vi "系统设置.vi"() -> ()   [LabVIEW 2016]
uses:
  <userlib>/_SmartBalloon/Balloon Generic/Aesthetics.ctl
  <vilib>/Utility/miscctls.llb/LVPointTypeDef.ctl
  <userlib>/_SmartBalloon/Balloon/Text Balloon.lvclass
  C:/Program Files (x86)/National Instruments/LabVIEW 2016/user.lib/_SmartBalloon/Balloon Generic/Balloon.lvclass
  <userlib>/_SmartBalloon/Balloon/Init Balloon.vi
  <vilib>/ptbypt/NI_PtbyPt.lvlib
  <vilib>/Utility/config.llb/NI_LVConfig.lvlib
  PLC/PLC.lvlib
  <userlib>/_SmartBalloon/API/SmartBalloon Library.lvclass
  <userlib>/_SmartBalloon/Balloon Generic/Balloon.lvclass
  API/WxMessage/wxpusher.lvlib
panel:
  out "最近一次启动时间":string
  in  "添加防火墙":bool
  in  "系统单次测试":bool
  in  "站点配置":bool
  in  "微信关注扫码":bool
  in  "updateconfiguration":T1={"主机"="27.154.58.30", "用户"="update", "密码"="std23506", "远程路径"="数据传输系统\\平台数据传输系统.exe", "下载文件名"="平台数据传输系统.exe", "软件版本"=""}
  in  "周期运行启动参数":T2
  in  "更新":bool
  in  "模块启用配置":bool
  in  "短信报警设置":bool
  in  "首页显示设置":bool
  in  "跨度核查":bool
  in  "空白核查":bool
  out "选项卡控件":enum32{"自由设定", "国标协议", "流量设定"}(tab)
  in  "24H周期设置":bool[](xcontrol)
  in  "多参数运行间隔":i16=4 min=1 max=24
  in  "运行间隔":i16=4 caption="湿化学运行间隔" min=1 max=24
  in  "流量阈值":dbl=4.0 min=1.0 max=24.0
  in  "时间阈值":u16=4 min=1 max=24
  in  "周期设置":enum16{"自由设定", "国标协议", "流量设定"}(ring)
  out "x = y?":bool
  in  "质控启动日期":string(combo)="关闭"
  in  "跨度核查时间":T3(ring)=enum."06H"
  in  "空白核查时间":T3(ring)=enum."02H"
  in  "输入密码":dbl
  out "布尔":bool
  in  "开机启动":bool caption="氨氮禁用"
  in  "运行模式":enum16{"维护模式", "常规模式", "应急模式", "质控模式"}(ring)
  # "注：周期设置分为自由设定和国标协议两种。\n1：选择自由设定情况下：运行间隔将不可选用并变灰色，周期设置可自由手动勾选\n2：选择国标协议情况下：周期时间将由运行间隔选择的时间决定，下方周期设置被禁用并无法手动勾选。\n3：选择流量设定情况下：瞬时流量连续超过流量阈值到达时间阈值设定值，仪器将自动开启测量。"
  # "质控频次："
  # "零点核查时间："
  # "跨度核查时间："
  # "启动周期设置"
  # "m3/S"
  # "秒"
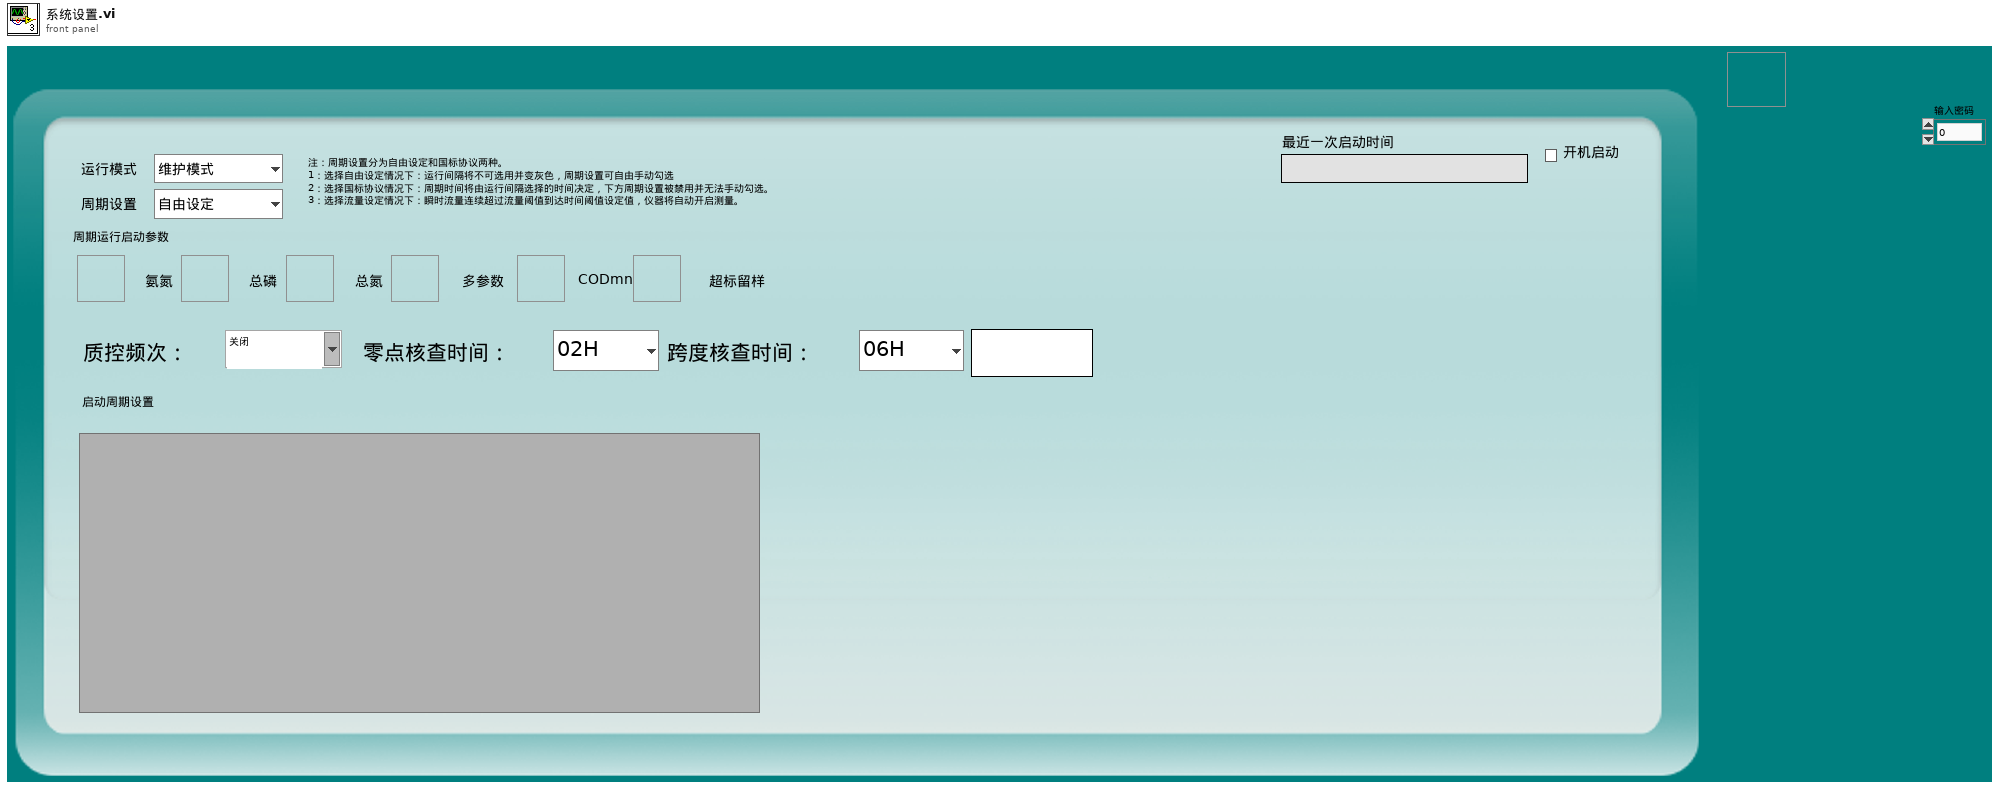
[diagram p1: front panel]
types:
  T1 = cluster{"主机":string, "用户":string, "密码":string, "远程路径":string, "下载文件名":string, "软件版本":string}
  T2 = cluster{"氨氮":bool, "总磷":bool, "总氮":bool, "多参数":bool, "CODmn":bool, "CODCr":bool, "超标留样":bool}
  T3 = enum16{"00H", "01H", "02H", "03H", "04H", "05H", "06H", "07H", "08H", "09H", "10H", "11H", "12H", "13H", "14H", "15H", "16H", "17H", "18H", "19H", "20H", "21H", "22H", "23H", "关闭"}
  T4 = enum16{"启动测量", "标样核查", "零点核查", "跨度核查", "空白测试", "平行样测试", "加标回收", "空白校准", "标样校准", "初始化（清洗）", "停止测试", "仪器重启", "校时", "模式设置", "测量间隔设置"}
  T5 = cluster{"参数启用":cluster{"氨氮":bool, "总磷":bool, "总氮":bool, "多参数":bool, "CODMn":bool, "CODcr":bool, "超标留样":bool}}
  T6 = typedef "LVPointTypeDef.ctl" = cluster{"Horizontal":i16, "Vertical":i16}
  T7 = enum32{"Bad", "Idle", "Run top level", "Running"}
  T8 = typedef "Balloon Engine.lvlib/Balloon.lvclass/Aesthetics.ctl" = cluster{"Colors":cluster{"Font Color":u32, "Panel Color":u32}, "Display Time (ms)":i32}
  T9 = cluster{"运行模式":enum16{"维护模式", "常规模式", "应急模式", "质控模式"}, "质控频次":enum16{"关闭", "每天", "星期一", "星期二", "星期三", "星期四", "星期五", "星期六", "星期日"}, "空白核查时间":u16, "跨度核查时间":u16, "24H周期设置":bool[]}
  T10 = typedef "LVDateTimeRec.ctl" = cluster{"秒数的小数部分":dbl, "秒":i32, "分":i32, "时":i32, "日":i32, "月":i32, "年":i32, "天数（周）":i32, "天数（年）":i32, "DST":i32}
  T11 = enum32{"Invalid", "Standard", "Closed", "Hidden", "Minimized", "Maximized"}
  T12 = typedef "NI_LVConfig.lvlib/Config Data RefNum.ctl" = refnum<k1>
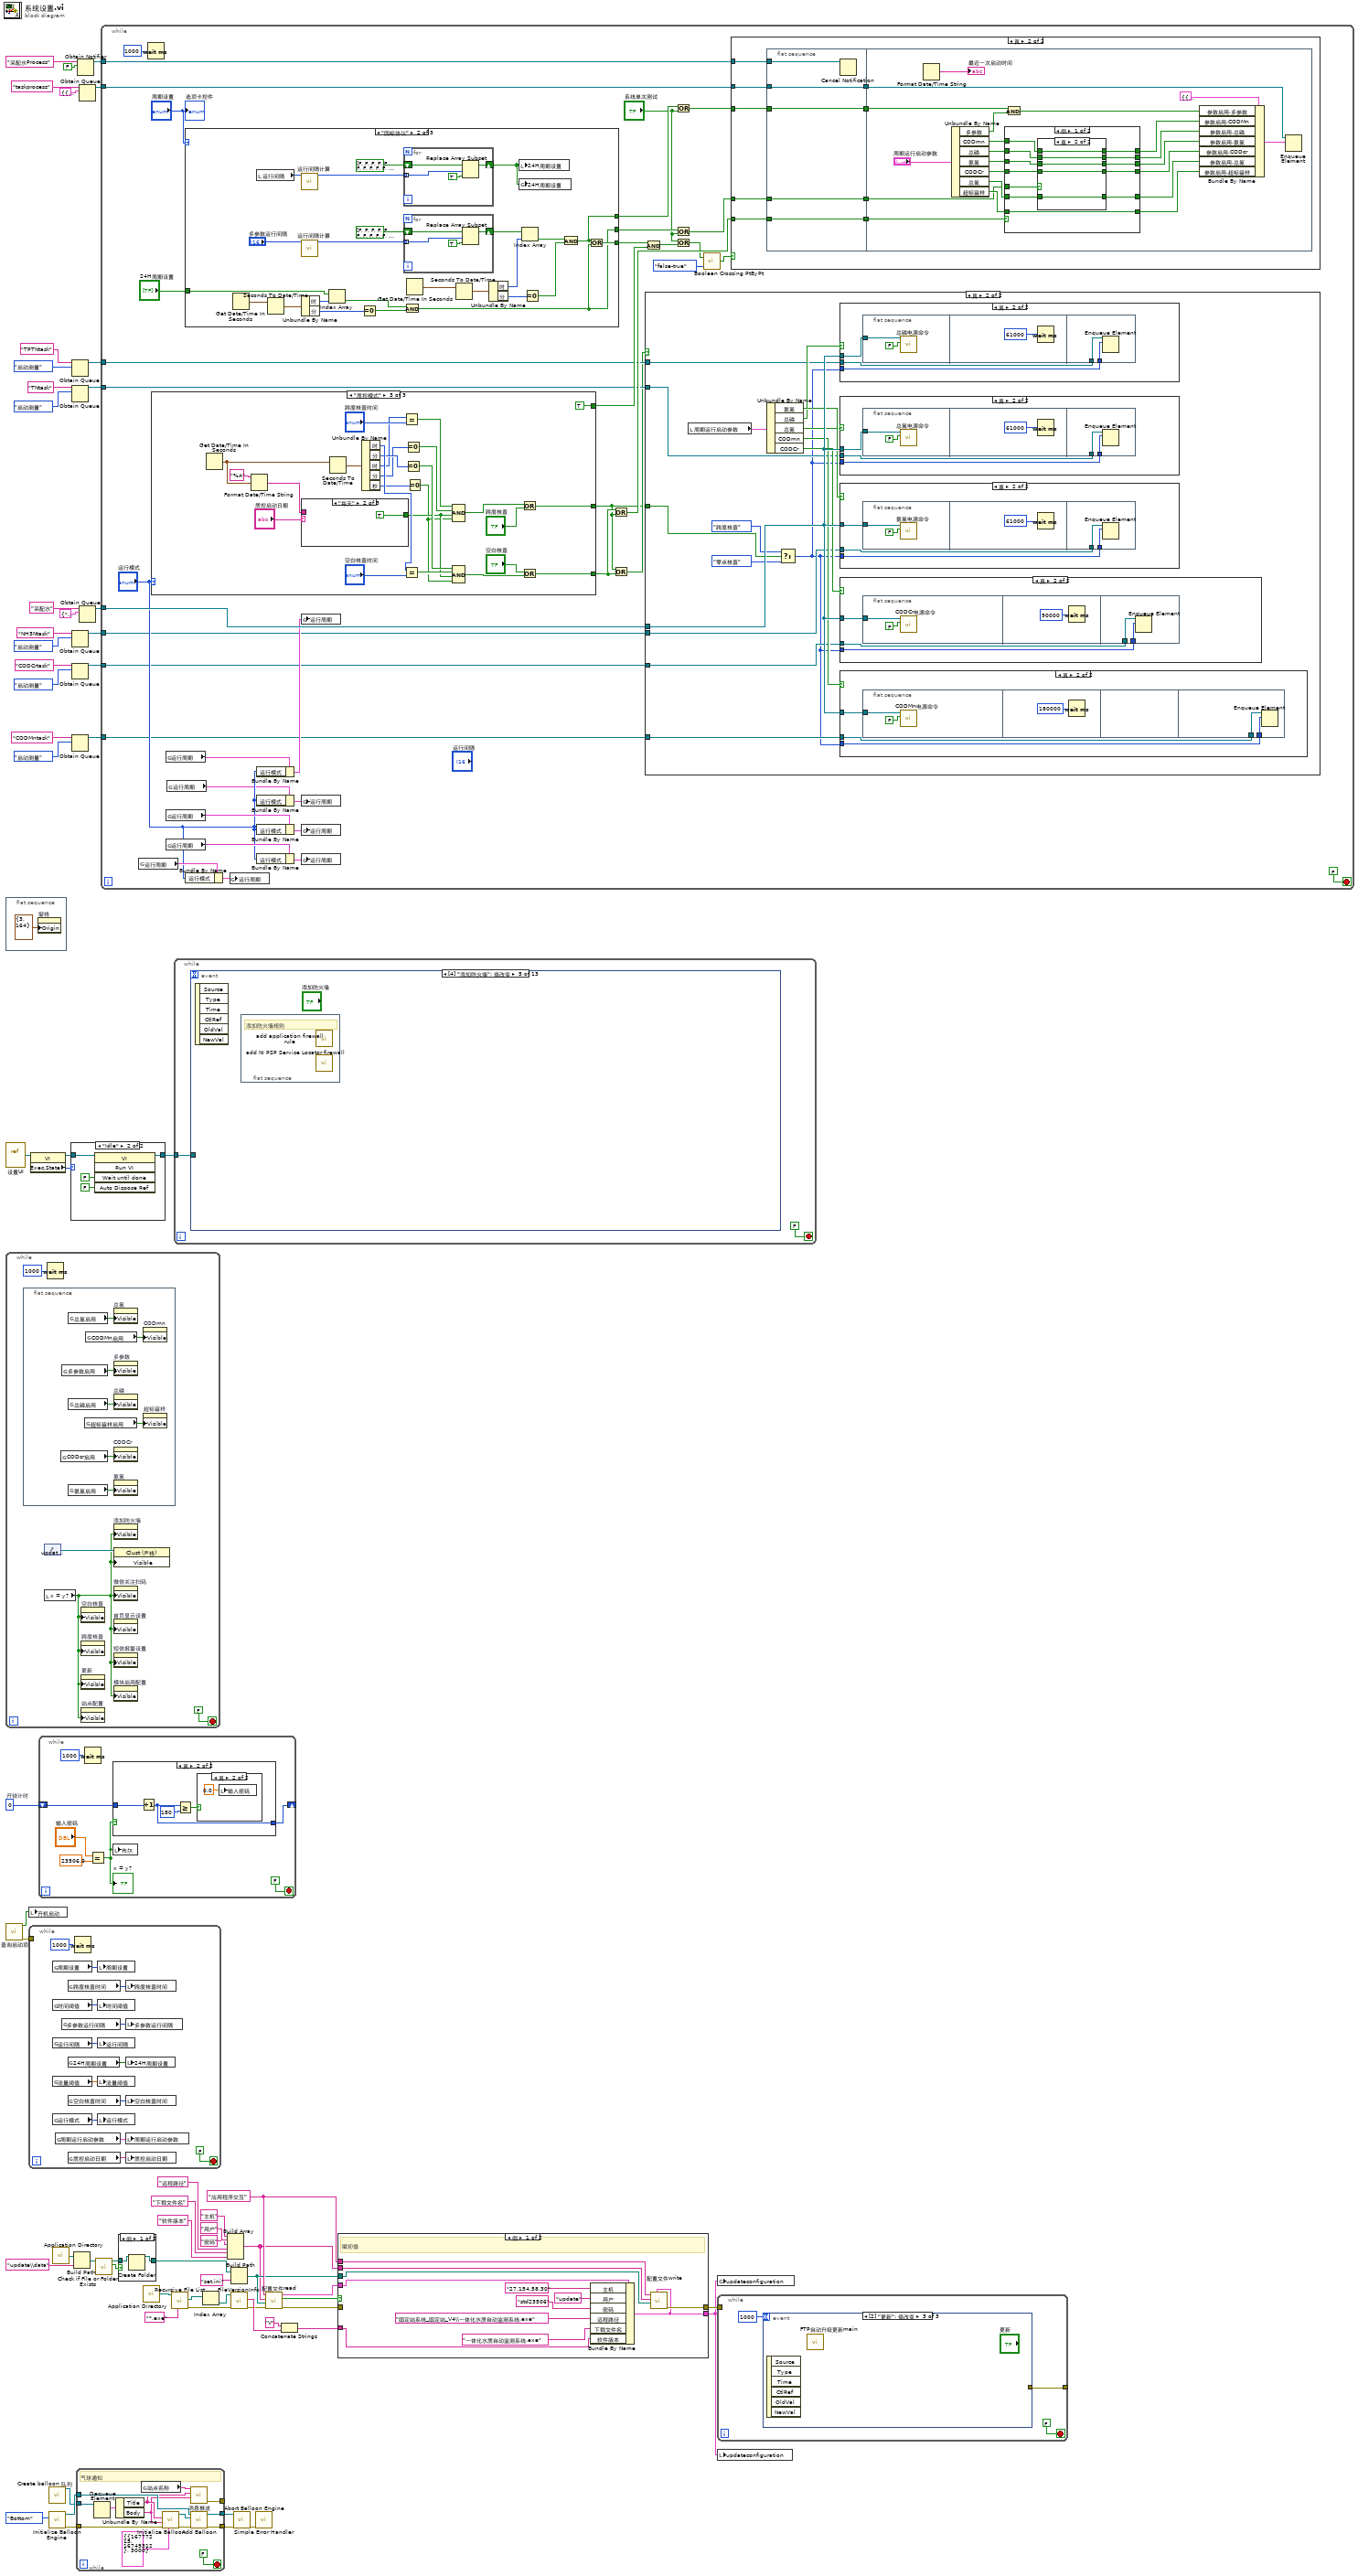
[diagram p0: block diagram]
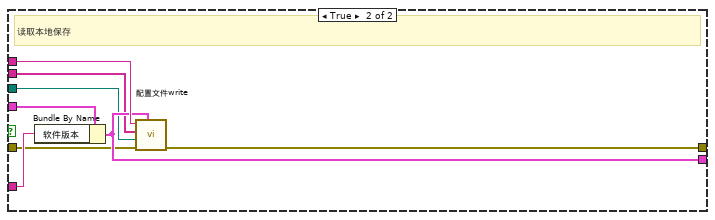
[diagram p3: hidden frame]
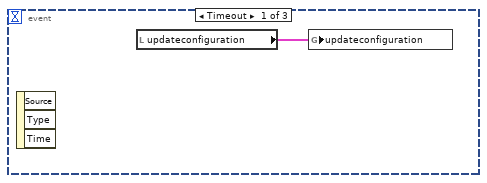
[diagram p4: hidden frame]
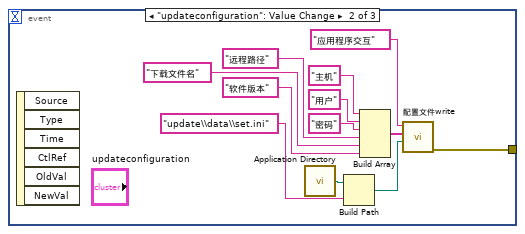
[diagram p5: hidden frame]
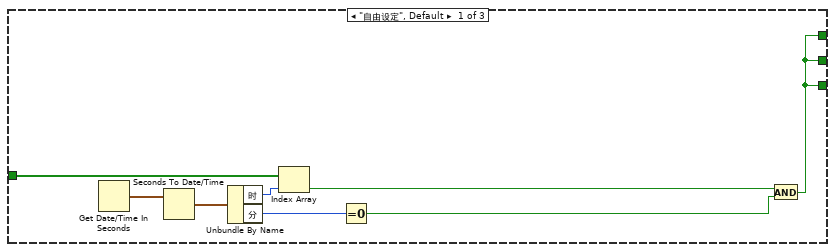
[diagram p9: hidden frame]
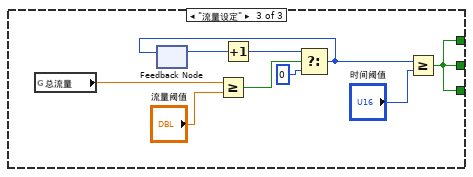
[diagram p10: hidden frame]
diagram:
  w53 = "应用程序交互" ("section")
  w64 = u32 0  # 开锁计时
  n1 = flat-sequence {
    frame #0 {
      n2 = property on="窗格" class="Pane"("Origin"=T6 {"Horizontal"=3, "Vertical"=164} ("原点")) -> ()  [unwired: 2 in, 2 out]
    }
  }
  n3 = vi-ref "设置UI.vi"() -> (w60:refnum<vi>)
  n4 = while {
    stop <- FALSE stop-if-true
    n5 = flat-sequence {
      frame #0 {
        n6 = global read "系统设置全局变量.vi" "CODcr启用"() -> (w76:bool)
        n7 = global read "系统设置全局变量.vi" "多参数启用"() -> (w77:bool)
        n8 = global read "系统设置全局变量.vi" "总氮启用"() -> (w79:bool)
        n9 = global read "系统设置全局变量.vi" "总磷启用"() -> (w75:bool)
        n10 = global read "系统设置全局变量.vi" "氨氮启用"() -> (w80:bool)
        n11 = global read "系统设置全局变量.vi" "超标留样启用"() -> (w74:bool)
        n12 = global read "系统设置全局变量.vi" "CODMn启用"() -> (w78:bool)
        n13 = property on="总氮" class="Bool (严格)"("Visible"=w79) -> ()  [unwired: 2 in, 2 out]
        n14 = property on="多参数" class="Bool (严格)"("Visible"=w77) -> ()  [unwired: 2 in, 2 out]
        n15 = property on="总磷" class="Bool (严格)"("Visible"=w75) -> ()  [unwired: 2 in, 2 out]
        n16 = property on="CODCr" class="Bool (严格)"("Visible"=w76) -> ()  [unwired: 2 in, 2 out]
        n17 = property on="氨氮" class="Bool (严格)"("Visible"=w80) -> ()  [unwired: 2 in, 2 out]
        n18 = property on="CODmn" class="Bool (严格)"("Visible"=w78) -> ()  [unwired: 2 in, 2 out]
        n19 = property on="超标留样" class="Bool (严格)"("Visible"=w74) -> ()  [unwired: 2 in, 2 out]
      }
    }
    n20 = control-ref of="updateconfiguration"() -> (w71:refnum<vi>)
    n21 = local read "x = y?"() -> (w70:bool)
    n22 = Wait (ms)(milliseconds to wait=u32 1000 ("等待时间（毫秒）")) -> ()  [unwired: 1 out]
    n23 = property on="空白核查" class="Bool"("Visible"=w70) -> ()  [unwired: 2 in, 2 out]
    n24 = property on="跨度核查" class="Bool"("Visible"=w70) -> ()  [unwired: 2 in, 2 out]
    n25 = property on="更新" class="Bool"("Visible"=w70) -> ()  [unwired: 2 in, 2 out]
    n26 = property on="站点配置" class="Bool"("Visible"=w70) -> ()  [unwired: 2 in, 2 out]
    n27 = property on="添加防火墙" class="Bool"("Visible"=w70) -> ()  [unwired: 2 in, 2 out]
    n28 = property class="Clust (严格)"(reference=w71, "Visible"=w70) -> ()  [unwired: 1 in, 2 out]
    n29 = property on="微信关注扫码" class="Bool"("Visible"=w70) -> ()  [unwired: 2 in, 2 out]
    n30 = property on="首页显示设置" class="Bool"("Visible"=w70) -> ()  [unwired: 2 in, 2 out]
    n31 = property on="短信报警设置" class="Bool"("Visible"=w70) -> ()  [unwired: 2 in, 2 out]
    n32 = property on="模块启用配置" class="Bool"("Visible"=w70) -> ()  [unwired: 2 in, 2 out]
  }
  n33 = call "查询启动项.vi"() -> ("error out"=w56:errorcluster, "包含启动项"=w65:bool)  [unwired: 9 in, 1 out]
  n34 = local write "开机启动"(w65) -> ()
  n35 = while {
    tunnel: w56 -> [_]
    stop <- FALSE stop-if-true
    n36 = global read "系统设置全局变量.vi" "周期设置"() -> (w87:enum16{"自由设定", "国标协议", "流量设定"})
    n37 = global read "系统设置全局变量.vi" "时间阈值"() -> (w83:u16)
    n38 = global read "系统设置全局变量.vi" "运行间隔"() -> (w86:i16)
    n39 = global read "系统设置全局变量.vi" "流量阈值"() -> (w84:dbl)
    n40 = global read "系统设置全局变量.vi" "运行模式"() -> (w85:enum16{"维护模式", "常规模式", "应急模式", "质控模式"})
    n41 = global read "系统设置全局变量.vi" "周期运行启动参数"() -> (w82:T2)
    n42 = global read "系统设置全局变量.vi" "多参数运行间隔"() -> (w81:i16)
    n43 = global read "系统设置全局变量.vi" "跨度核查时间"() -> (w88:u16)
    n44 = global read "系统设置全局变量.vi" "24H周期设置"() -> (w91:bool[])
    n45 = global read "系统设置全局变量.vi" "空白核查时间"() -> (w89:u16)
    n46 = global read "系统设置全局变量.vi" "质控启动日期"() -> (w90:string)
    n47 = Wait (ms)(milliseconds to wait=u32 1000 ("等待时间（毫秒）")) -> ()  [unwired: 1 out]
    n48 = local write "周期设置"(w87) -> ()
    n49 = local write "时间阈值"(w83) -> ()
    n50 = local write "运行间隔"(w86) -> ()
    n51 = local write "流量阈值"(w84) -> ()
    n52 = local write "运行模式"(w85) -> ()
    n53 = local write "跨度核查时间"(w88) -> ()
    n54 = local write "多参数运行间隔"(w81) -> ()
    n55 = local write "24H周期设置"(w91) -> ()
    n56 = local write "空白核查时间"(w89) -> ()
    n57 = local write "周期运行启动参数"(w82) -> ()
    n58 = local write "质控启动日期"(w90) -> ()
  }
  n59 = property class="VI"(reference=w60) -> (reference out=w58:refnum<vi>, "Exec.State"=w59:T7)  [unwired: 1 in, 1 out]
  n60 = while {
    shift-right: [w95] -> _
    shift-left: w64 -> [w96]
    stop <- FALSE stop-if-true
    n61 = Wait (ms)(milliseconds to wait=u32 1000 ("等待时间（毫秒）")) -> ()  [unwired: 1 out]
    n62 = Equal?(x="输入密码", y=23506.0) -> (x = y?=w94:bool)
    "x = y?" <- w94
    n63 = case shown="真" w94 {
      tunnel: w96 -> [_ w104]
      tunnel: [_ w103] -> w95
      frame False {
      }
      frame True {
        n64 = Increment(x=w104) -> (x+1=w103:u32)
        n65 = Greater Or Equal?(x=w103, y=u32 180) -> (x >= y?=w101:bool)
        n66 = case shown="真" w101 {
          frame False {
          }
          frame True {
            n67 = local write "输入密码"(0.0 ("输入密码")) -> ()
          }
        }
      }
    }
    n68 = local write "布尔"(w94) -> ()
  }
  n69 = call "Create balloon 队列.vi"() -> ("队列输出"=w19:refnum<queue>)  [unwired: 11 in]
  n70 = call <userlib>:"Initialize Balloon Engine.vi"("Balloon Direction"=enum16{"Top", "Bottom"}."Bottom" ("Balloon Position")) -> ("error out"=w21:errorcluster, "SmartBalloon Library.lvclass"=w24:refnum<class "SmartBalloon Library.lvclass">)  [unwired: 9 in]
  n71 = call <vilib>:"Application Directory.vi"() -> ("Application Directory"=w30:path)
  n72 = case shown="\"Idle\"" w59 {
    tunnel: w58 -> [w106 w110]
    tunnel: [w106 w109] -> w57
    frame "Bad", Default {
    }
    frame "Idle" {
      n73 = invoke class="VI" method="Run VI"(reference=w110, "Wait until done"=FALSE ("结束前等待"), "Auto Dispose Ref"=FALSE ("自动销毁引用")) -> (reference out=w109:refnum<vi>)  [unwired: 2 in, 4 out]
    }
  }
  n74 = Obtain Queue(name (unnamed)="TPTNtask" ("名称（未命名）"), element data type=T4."启动测量" ("控制命令")) -> (queue out=w5:refnum<queue>)  [unwired: 3 in, 2 out]
  n75 = Obtain Queue(name (unnamed)="TNtask" ("名称（未命名）"), element data type=T4."启动测量" ("控制命令")) -> (queue out=w3:refnum<queue>)  [unwired: 3 in, 2 out]
  n76 = Obtain Queue(name (unnamed)="NH3Ntask" ("名称（未命名）"), element data type=T4."启动测量" ("控制命令")) -> (queue out=w4:refnum<queue>)  [unwired: 3 in, 2 out]
  n77 = Obtain Queue(name (unnamed)="CODCrtask" ("名称（未命名）"), element data type=T4."启动测量" ("控制命令")) -> (queue out=w2:refnum<queue>)  [unwired: 3 in, 2 out]
  n78 = Obtain Queue(name (unnamed)="CODMntask" ("名称（未命名）"), element data type=T4."启动测量" ("控制命令")) -> (queue out=w1:refnum<queue>)  [unwired: 3 in, 2 out]
  n79 = Build Path(base path=w30, name or relative path="update\\data" ("名称或相对路径")) -> (appended path=w31:path)
  n80 = while {
    tunnel: w24 -> [w124]
    tunnel: [w123] -> w23
    tunnel: [w121] -> w22
    tunnel: w21 -> [w122]
    tunnel: w19 -> [w119]
    tunnel: [w112] -> _
    stop <- FALSE stop-if-true
    # "气球通知"
    n81 = Dequeue Element(queue=w119) -> (element=w115:cluster{"Title":string, "Body":string})  [unwired: 2 in, 3 out]
    n82 = Unbundle By Name(w115) -> ("Title"=w114:string, "Body"=w113:string)
    n83 = global read "系统设置全局变量.vi" "站点名称"() -> (w111:string)
    n84 = call-poly <userlib>:"Initialize Balloon.vi"("Aesthetics"=T8 {"Colors"={"Font Color"=16777215, "Panel Color"=16749312}, "Display Time (ms)"=3000}, "error in (no error)"=w122, "Body"=w113, "Title"=w114) -> ("error out"=w116:errorcluster, "Balloon out"=w118:refnum<class "Text Balloon.lvclass">)  [unwired: 6 in]
    n85 = call "消息推送.vi"("分析"=w113, "内容"=w114, "站点"=w111) -> ("error out"=w112:errorcluster)  [unwired: 8 in]
    n86 = call <userlib>:"Add Balloon.vi"("error in (no error)"=w116, "Next Balloon"=w118, "SmartBalloon Engine Reference"=w124) -> ("error out"=w121:errorcluster, "SmartBalloon Engine Reference out"=w123:refnum<class "SmartBalloon Library.lvclass">)  [unwired: 7 in]
  }
  n87 = Obtain Notifier(name (unnamed)="采配水Process" ("名称（未命名）"), notification data type=FALSE) -> (notifier out=w66:refnum<notifier>)  [unwired: 2 in, 2 out]
  n88 = Obtain Queue(name (unnamed)="taskprocess" ("名称（未命名）"), element data type=T5 {"参数启用"={"氨氮"=FALSE, "总磷"=FALSE, "总氮"=FALSE, "多参数"=FALSE, "CODMn"=FALSE, "CODcr"=FALSE, "超标留样"=FALSE}} ("参数")) -> (queue out=w16:refnum<queue>)  [unwired: 3 in, 2 out]
  n89 = Obtain Queue(name (unnamed)="采配水" ("名称（未命名）"), element data type=cluster{"命令":string, "数据":variant} {"命令"="", "数据"=variant}) -> (queue out=w61:refnum<queue>)  [unwired: 3 in, 2 out]
  n90 = call <vilib>:"Check if File or Folder Exists.vi"("path"=w31) -> ("file or folder exists?"=w32:bool, "dup path"=w33:path)  [unwired: 8 in, 1 out]
  n91 = while {
    tunnel: w66 -> [w160]
    tunnel: w61 -> [w157]
    tunnel: w16 -> [w133]
    tunnel: w5 -> [w132]
    tunnel: w4 -> [w131]
    tunnel: w3 -> [w130]
    tunnel: w2 -> [w129]
    tunnel: w1 -> [w128]
    stop <- FALSE stop-if-true
    n92 = global read "总磷总氮断电保存全局变量.vi" "运行周期"() -> (w150:T9)
    n93 = Wait (ms)(milliseconds to wait=u32 1000 ("等待时间（毫秒）")) -> ()  [unwired: 1 out]
    n94 = case shown="\"质控模式\"" "运行模式" {
      tunnel: [_ _ w322] -> w125
      tunnel: [_ _ w326] -> w126
      tunnel: [_ TRUE TRUE] -> w154
      frame "维护模式", Default {
      }
      frame "常规模式" {
      }
      frame "质控模式" {
        n95 = Get Date/Time In Seconds() -> (seconds since 1Jan1904=w333:timestamp)
        n96 = Format Date/Time String(time format string (%c)="%A" ("时间格式字符串(%c)"), seconds (now)=w333) -> (date/time string=w331:string)  [unwired: 1 in]
        n97 = case shown="\"每天\"" "质控启动日期" {
          selector: "质控启动日期" -> [w349 _ _]
          tunnel: [w348 TRUE FALSE] -> w334
          tunnel: w331 -> [w347 _ _]
          frame "星期二", "星期六", "星期日", "星期三", "星期四", "星期五", "星期一" {
            n98 = Equal?(x=w347, y=w349) -> (x = y?=w348:bool)
          }
          frame "每天" {
          }
          frame "关闭", Default {
          }
        }
        n99 = Seconds To Date/Time(time stamp (now)=w333) -> (date time rec=w346:T10)  [unwired: 1 in]
        n100 = Unbundle By Name(w346) -> ("时"=w345:i32, "分"=w343:i32, "时"=w339:i32, "分"=w338:i32, "秒"=w330:i32)
        n101 = Equal?(x=w339, y="跨度核查时间") -> (x = y?=w337:bool)
        n102 = Equal?(x=w345, y="空白核查时间") -> (x = y?=w342:bool)
        n103 = Equal To 0?(x=w338) -> (x = 0?=w336:bool)
        n104 = Equal To 0?(x=w343) -> (x = 0?=w341:bool)
        n105 = Equal To 0?(x=w330) -> (x = 0?=w329:bool)
        n106 = Compound Arithmetic op=AND ("复合运算")(w337, w336, w334, w329) -> (w324:bool)
        n107 = Compound Arithmetic op=AND ("复合运算")(w341, w342, w334, w329) -> (w327:bool)
        n108 = Or(x=w324, y="跨度核查") -> (x .or. y?=w322:bool)
        n109 = Or(x="空白核查", y=w327) -> (x .or. y?=w326:bool)
      }
    }
    n110 = global read "总磷总氮断电保存全局变量.vi" "运行周期"() -> (w140:T9)
    n111 = global read "总磷总氮断电保存全局变量.vi" "运行周期"() -> (w146:T9)
    n112 = global read "总磷总氮断电保存全局变量.vi" "运行周期"() -> (w148:T9)
    n113 = global read "CODMn断电保存全局变量.vi" "运行周期"() -> (w142:T9)
    n114 = case shown="\"国标协议\"" "周期设置" {
      tunnel: [w163 w173 w203] -> w153
      tunnel: "24H周期设置" -> [w164 w184 _]
      tunnel: [w163 w172 w203] -> w137
      tunnel: [w163 w171 w203] -> w138
      frame "自由设定", Default {
        n115 = Get Date/Time In Seconds() -> (seconds since 1Jan1904=w165:timestamp)
        n116 = Seconds To Date/Time(time stamp (now)=w165) -> (date time rec=w166:T10)  [unwired: 1 in]
        n117 = Unbundle By Name(w166) -> ("时"=w169:i32, "分"=w167:i32)
        n118 = Index Array(array=w164, index=w169) -> (element=w170:bool)
        n119 = Equal To 0?(x=w167) -> (x = 0?=w168:bool)
        n120 = And(x=w170, y=w168) -> (x .and. y?=w163:bool)
      }
      frame "国标协议" {
        n121 = Get Date/Time In Seconds() -> (seconds since 1Jan1904=w185:timestamp)
        n122 = local read "运行间隔"() -> (w194:i16)
        n123 = Seconds To Date/Time(time stamp (now)=w185) -> (date time rec=w186:T10)  [unwired: 1 in]
        n124 = call "运行间隔计算.vi"("运行周期"=w194) -> ("数组"=w193:i32[])  [unwired: 10 in]
        n125 = call "运行间隔计算.vi"("运行周期"="多参数运行间隔") -> ("数组"=w176:i32[])  [unwired: 10 in]
        n126 = Unbundle By Name(w186) -> ("时"=w189:i32, "分"=w187:i32)
        n127 = Index Array(array=w184, index=w189) -> (element=w190:bool)
        n128 = Equal To 0?(x=w187) -> (x = 0?=w188:bool)
        n129 = for {
          tunnel: w193 -> [w201] mode=indexing
          shift-right: [w199] -> w191
          shift-left: bool[] [FALSE, FALSE, FALSE, FALSE, FALSE, FALSE, FALSE, FALSE, FALSE, FALSE, FALSE, FALSE, FALSE, FALSE, FALSE, FALSE, FALSE, FALSE, FALSE, FALSE, FALSE, FALSE, FALSE, FALSE] ("24H周期设置") -> [w202]
          n130 = Replace Array Subset(array=w202, new element=TRUE ("新元素/子数组"), index=w201) -> (w199:bool[])
        }
        n131 = for {
          tunnel: w176 -> [w197] mode=indexing
          shift-right: [w195] -> w174
          shift-left: bool[] [FALSE, FALSE, FALSE, FALSE, FALSE, FALSE, FALSE, FALSE, FALSE, FALSE, FALSE, FALSE, FALSE, FALSE, FALSE, FALSE, FALSE, FALSE, FALSE, FALSE, FALSE, FALSE, FALSE, FALSE] ("24H周期设置") -> [w198]
          n132 = Replace Array Subset(array=w198, new element=TRUE ("新元素/子数组"), index=w197) -> (w195:bool[])
        }
        n133 = And(x=w190, y=w188) -> (x .and. y?=w171:bool)
        n134 = Get Date/Time In Seconds() -> (seconds since 1Jan1904=w183:timestamp)
        n135 = Seconds To Date/Time(time stamp (now)=w183) -> (date time rec=w182:T10)  [unwired: 1 in]
        n136 = Unbundle By Name(w182) -> ("时"=w179:i32, "分"=w181:i32)
        n137 = local write "24H周期设置"(w191) -> ()
        n138 = global write "系统设置全局变量.vi" "24H周期设置"(w191) -> ()
        n139 = Index Array(array=w174, index=w179) -> (element=w178:bool)
        n140 = Equal To 0?(x=w181) -> (x = 0?=w180:bool)
        n141 = And(x=w178, y=w180) -> (x .and. y?=w172:bool)
        n142 = Or(x=w172, y=w171) -> (x .or. y?=w173:bool)
      }
      frame "流量设定" {
        n143 = global read "流量计全局变量.vi" "总流量"() -> (w211:dbl)
        n144 = feedback #1() -> (w208:i16)  [unwired: 1 in]
        n145 = Greater Or Equal?(x=w211, y="流量阈值") -> (x >= y?=w206:bool)
        n146 = Increment(x=w208) -> (x+1=w207:i16)
        n147 = Select(t=w207, s=w206, f=i16 0) -> (s? t:f=w205:i16)
        n148 = feedback-in #1(w205) -> ()
        n149 = Greater Or Equal?(x=w205, y="时间阈值") -> (x >= y?=w203:bool)
      }
    }
    n150 = Bundle By Name(cluster=w150, "运行模式"="运行模式") -> (w149:T9)
    n151 = global write "总磷总氮断电保存全局变量.vi" "运行周期"(w149) -> ()
    n152 = Bundle By Name(cluster=w140, "运行模式"="运行模式") -> (w139:T9)
    n153 = Bundle By Name(cluster=w142, "运行模式"="运行模式") -> (w141:T9)
    n154 = Bundle By Name(cluster=w146, "运行模式"="运行模式") -> (w145:T9)
    n155 = Bundle By Name(cluster=w148, "运行模式"="运行模式") -> (w147:T9)
    n156 = global write "总磷总氮断电保存全局变量.vi" "运行周期"(w139) -> ()
    n157 = global write "CODMn断电保存全局变量.vi" "运行周期"(w141) -> ()
    n158 = global write "总磷总氮断电保存全局变量.vi" "运行周期"(w145) -> ()
    n159 = global write "总磷总氮断电保存全局变量.vi" "运行周期"(w147) -> ()
    n160 = Or(x=w126, y=w125) -> (x .or. y?=w151:bool)
    n161 = Or(x=w125, y=w126) -> (x .or. y?=w127:bool)
    n162 = And(x=w153, y=w154) -> (x .and. y?=w152:bool)
    n163 = case shown="真" w127 {
      tunnel: w157 -> [_ w227]
      tunnel: w132 -> [_ w220]
      tunnel: w131 -> [_ w219]
      tunnel: w130 -> [_ w218]
      tunnel: w129 -> [_ w217]
      tunnel: w128 -> [_ w216]
      tunnel: w125 -> [_ w215]
      frame False {
      }
      frame True {
        n164 = local read "周期运行启动参数"() -> (w226:T2)
        n165 = Unbundle By Name(w226) -> ("氨氮"=w223:bool, "总磷"=w221:bool, "总氮"=w222:bool, "CODmn"=w224:bool, "CODCr"=w225:bool)
        n166 = Select(t=T4."跨度核查" ("元素"), s=w215, f=T4."零点核查" ("元素")) -> (s? t:f=w212:T4)
        n167 = case shown="真" w221 {
          tunnel: w227 -> [_ w230]
          tunnel: w220 -> [_ w229]
          tunnel: w212 -> [_ w228]
          frame False {
          }
          frame True {
            n168 = flat-sequence {
              tunnel: w230 -> [w232]
              tunnel: w229 -> [w235]
              tunnel: w228 -> [w234]
              frame #0 {
                n169 = call "总磷电源命令.vi"("通电/断电"=FALSE, "队列"=w232) -> ()  [unwired: 9 in, 1 out]
              }
              frame #1 {
                n170 = Wait (ms)(milliseconds to wait=u32 61000 ("等待时间（毫秒）")) -> ()  [unwired: 1 out]
              }
              frame #2 {
                n171 = Enqueue Element(queue=w235, element=w234) -> ()  [unwired: 2 in, 3 out]
              }
            }
          }
        }
        n172 = case shown="真" w222 {
          tunnel: w227 -> [_ w254]
          tunnel: w218 -> [_ w253]
          tunnel: w212 -> [_ w252]
          frame False {
          }
          frame True {
            n173 = flat-sequence {
              tunnel: w254 -> [w256]
              tunnel: w253 -> [w259]
              tunnel: w252 -> [w258]
              frame #0 {
                n174 = call "总氮电源命令.vi"("通电/断电"=FALSE, "队列"=w256) -> ()  [unwired: 9 in, 1 out]
              }
              frame #1 {
                n175 = Wait (ms)(milliseconds to wait=u32 61000 ("等待时间（毫秒）")) -> ()  [unwired: 1 out]
              }
              frame #2 {
                n176 = Enqueue Element(queue=w259, element=w258) -> ()  [unwired: 2 in, 3 out]
              }
            }
          }
        }
        n177 = case shown="真" w223 {
          tunnel: w227 -> [_ w262]
          tunnel: w219 -> [_ w261]
          tunnel: w212 -> [_ w260]
          frame False {
          }
          frame True {
            n178 = flat-sequence {
              tunnel: w262 -> [w263]
              tunnel: w261 -> [w267]
              tunnel: w260 -> [w266]
              frame #0 {
                n179 = call "氨氮电源命令.vi"("通电/断电"=FALSE, "队列"=w263) -> ()  [unwired: 9 in, 1 out]
              }
              frame #1 {
                n180 = Wait (ms)(milliseconds to wait=u32 61000 ("等待时间（毫秒）")) -> ()  [unwired: 1 out]
              }
              frame #2 {
                n181 = Enqueue Element(queue=w267, element=w266) -> ()  [unwired: 2 in, 3 out]
              }
            }
          }
        }
        n182 = case shown="真" w225 {
          tunnel: w227 -> [_ w238]
          tunnel: w217 -> [_ w237]
          tunnel: w212 -> [_ w236]
          frame False {
          }
          frame True {
            n183 = flat-sequence {
              tunnel: w238 -> [w239]
              tunnel: w237 -> [w243]
              tunnel: w236 -> [w242]
              frame #0 {
                n184 = call "CODCr电源命令.vi"("通电/断电"=FALSE, "队列"=w239) -> ()  [unwired: 9 in, 1 out]
              }
              frame #1 {
                n185 = Wait (ms)(milliseconds to wait=u32 90000 ("等待时间（毫秒）")) -> ()  [unwired: 1 out]
              }
              frame #2 {
                n186 = Enqueue Element(queue=w243, element=w242) -> ()  [unwired: 2 in, 3 out]
              }
            }
          }
        }
        n187 = case shown="真" w224 {
          tunnel: w227 -> [_ w246]
          tunnel: w216 -> [_ w245]
          tunnel: w212 -> [_ w244]
          frame False {
          }
          frame True {
            n188 = flat-sequence {
              tunnel: w246 -> [w247]
              tunnel: w245 -> [w251]
              tunnel: w244 -> [w250]
              frame #0 {
                n189 = call "CODMn电源命令.vi"("通电/断电"=FALSE, "队列"=w247) -> ()  [unwired: 9 in, 1 out]
              }
              frame #1 {
                n190 = Wait (ms)(milliseconds to wait=u32 180000 ("等待时间（毫秒）")) -> ()  [unwired: 1 out]
              }
              frame #2 {
              }
              frame #3 {
                n191 = Enqueue Element(queue=w251, element=w250) -> ()  [unwired: 2 in, 3 out]
              }
            }
          }
        }
      }
    }
    n192 = Or(x=w137, y="系统单次测试") -> (x .or. y?=w135:bool)
    n193 = Or(x=w138, y="系统单次测试") -> (x .or. y?=w136:bool)
    n194 = Or(x="系统单次测试", y=w152) -> (x .or. y?=w144:bool)
    n195 = call <vilib>:"Boolean Crossing PtByPt.vi"("direction"=enum16{"either", "false-true", "true-false"}."false-true", "input"=w144) -> ("crossing"=w158:bool)  [unwired: 1 in]
    n196 = case shown="真" w158 {
      tunnel: w160 -> [_ w276]
      tunnel: w151 -> [_ w270]
      tunnel: w135 -> [_ w274]
      tunnel: w136 -> [_ w272]
      tunnel: w133 -> [_ w268]
      frame False {
      }
      frame True {
        n197 = flat-sequence {
          tunnel: w276 -> [w281]
          tunnel: [w280] -> w275
          tunnel: w274 -> [w280]
          tunnel: [w279] -> w273
          tunnel: w272 -> [w279]
          tunnel: [w278] -> w271
          tunnel: w270 -> [w278]
          tunnel: [w277] -> w269
          tunnel: w268 -> [w277]
          tunnel: w275 -> [w286]
          tunnel: w273 -> [w284]
          tunnel: w271 -> [w285]
          tunnel: w269 -> [w283]
          frame #0 {
            n198 = Cancel Notification(0:w281) -> ()  [unwired: 1 in, 3 out]
          }
          frame #1 {
            n199 = Format Date/Time String() -> (date/time string=→"最近一次启动时间":string)  [unwired: 3 in]
            n200 = Unbundle By Name("周期运行启动参数") -> ("多参数"=w295:bool, "CODmn"=w296:bool, "总磷"=w297:bool, "氨氮"=w298:bool, "CODCr"=w299:bool, "总氮"=w293:bool, "超标留样"=w292:bool)
            n201 = case shown="假" w285 {
              tunnel: [w314 _] -> w303
              tunnel: [w312 _] -> w302
              tunnel: [w308 _] -> w301
              tunnel: [w309 _] -> w300
              tunnel: w299 -> [w307 _]
              tunnel: w298 -> [w310 _]
              tunnel: w297 -> [w311 _]
              tunnel: w296 -> [w313 _]
              tunnel: [w305 _] -> w294
              tunnel: w293 -> [w306 _]
              tunnel: w292 -> [w304 _]
              tunnel: [w304 _] -> w291
              tunnel: w284 -> [w315 _]
              frame False {
                n202 = case shown="真" w315 {
                  tunnel: [_ w320] -> w314
                  tunnel: w313 -> [_ w320]
                  tunnel: [_ w319] -> w312
                  tunnel: w311 -> [_ w319]
                  tunnel: [_ w318] -> w309
                  tunnel: w310 -> [_ w318]
                  tunnel: [_ w317] -> w308
                  tunnel: w307 -> [_ w317]
                  tunnel: [_ w316] -> w305
                  tunnel: w306 -> [_ w316]
                  frame False {
                  }
                  frame True {
                  }
                }
              }
              frame True {
              }
            }
            n203 = And(x=w286, y=w295) -> (x .and. y?=w290:bool)
            n204 = Bundle By Name(cluster=T5 {"参数启用"={"氨氮"=FALSE, "总磷"=FALSE, "总氮"=FALSE, "多参数"=FALSE, "CODMn"=FALSE, "CODcr"=FALSE, "超标留样"=FALSE}} ("参数"), "参数启用.多参数"=w290, "参数启用.CODMn"=w303, "参数启用.总磷"=w302, "参数启用.氨氮"=w300, "参数启用.CODcr"=w301, "参数启用.总氮"=w294, "参数启用.超标留样"=w291) -> (w288:T5)
            n205 = Enqueue Element(queue=w283, element=w288) -> ()  [unwired: 2 in, 3 out]
          }
        }
      }
    }
    "选项卡控件" <- "周期设置"
  }
  n206 = case shown="假" w32 {
    tunnel: w33 -> [w353 w354]
    tunnel: [w352 w354] -> w28
    frame False {
      n207 = Create Folder(path (use dialog)=w353) -> (created path=w352:path)  [unwired: 2 in, 2 out]
    }
    frame True {
    }
  }
  n208 = call <vilib>:"Application Directory.vi"() -> ("Application Directory"=w48:path)
  n209 = call <vilib>:"Recursive File List.vi"("pattern"="*.exe", "Folder Path"=w48) -> ("error out"=w45:errorcluster, "All Files in Dir"=w47:path[])  [unwired: 5 in, 3 out]
  n210 = while {
    tunnel: w57 -> [w355]
    stop <- FALSE stop-if-true
    n211 = event shown="[4] \"添加防火墙\": 值改变" {
      selector: _ -> [_ _ _ _ _ _ _ _ _ _ _ _ _]
      dyn-events: _ -> [_ _ _ _ _ _ _ _ _ _ _ _ _]
      timeout: _ -> [_ _ _ _ _ _ _ _ _ _ _ _ _]
      tunnel: w355 -> [_ _ _ _ _ _ _ _ _ w405 _ _ _]
      event Timeout {
        n212 = event-data() -> ()  [unwired: 1 in, 3 out]
      }
      event "模块启用配置": Value Change {
        n213 = event-data() -> ()  [unwired: 1 in, 6 out]
        n214 = call "模块启用配置框.vi"() -> ()  [unwired: 12 in]
      }
      event "24H周期设置", "运行模式", "质控启动日期", "空白核查时间", "跨度核查时间", "运行间隔", "周期设置", "流量阈值", "时间阈值", "周期运行启动参数", "多参数运行间隔": Value Change {
        n215 = event-data() -> ()  [unwired: 1 in, 6 out]
        n216 = flat-sequence {
          frame #0 {
            n217 = local read "周期设置"() -> (w361:enum16{"自由设定", "国标协议", "流量设定"})
            n218 = local read "流量阈值"() -> (w359:dbl)
            n219 = local read "运行模式"() -> (w367:enum16{"维护模式", "常规模式", "应急模式", "质控模式"})
            n220 = local read "时间阈值"() -> (w360:u16)
            n221 = local read "运行间隔"() -> (w362:i16)
            n222 = local read "周期运行启动参数"() -> (w358:T2)
            n223 = local read "多参数运行间隔"() -> (w357:i16)
            n224 = local read "跨度核查时间"() -> (w363:T3)
            n225 = local read "24H周期设置"() -> (w366:bool[])
            n226 = local read "质控启动日期"() -> (w365:string)
            n227 = local read "空白核查时间"() -> (w364:T3)
            n228 = global write "系统设置全局变量.vi" "周期设置"(w361) -> ()
            n229 = global write "系统设置全局变量.vi" "流量阈值"(w359) -> ()
            n230 = global write "系统设置全局变量.vi" "运行模式"(w367) -> ()
            n231 = global write "系统设置全局变量.vi" "时间阈值"(w360) -> ()
            n232 = global write "系统设置全局变量.vi" "运行间隔"(w362) -> ()
            n233 = global write "系统设置全局变量.vi" "跨度核查时间"(w363) -> ()
            n234 = global write "系统设置全局变量.vi" "24H周期设置"(w366) -> ()
            n235 = global write "系统设置全局变量.vi" "质控启动日期"(w365) -> ()
            n236 = global write "系统设置全局变量.vi" "空白核查时间"(w364) -> ()
            n237 = global write "系统设置全局变量.vi" "多参数运行间隔"(w357) -> ()
            n238 = global write "系统设置全局变量.vi" "周期运行启动参数"(w358) -> ()
          }
          frame #1 {
            n239 = call <vilib>:"Application Directory.vi"() -> ("Application Directory"=w369:path)
            n240 = Build Path(base path=w369, name or relative path="data\\sys.ini" ("名称或相对路径")) -> (appended path=w368:path)
            n241 = call <vilib>:"Open Config Data.vi"("configuration file path"=w368) -> ("error out"=w378:errorcluster, "refnum"=w381:T12)  [unwired: 8 in, 1 out]
            n242 = vi-ref "系统设置全局变量.vi"() -> (w380:refnum<vi>)
            n243 = call <userlib>:"Write Panel to INI__ogtk.vi"("error in (no error)"=w378, "VI ref"=w380, "refnum"=w381) -> ("error out"=w377:errorcluster, "refnum out"=w379:T12)  [unwired: 7 in]
            n244 = call <vilib>:"Close Config Data.vi"("error in (no error)"=w377, "refnum"=w379) -> ("error out"=w372:errorcluster, "file path"=w371:path)  [unwired: 8 in]
            n245 = Open/Create/Replace File(file path (use dialog)=w371, error in=w372) -> (refnum out=w375:refnum<file>, error out=w376:errorcluster)  [unwired: 4 in, 1 out]
            n246 = Flush File(refnum=w375, error in=w376) -> (refnum out=w374:refnum<file>, error out=w373:errorcluster)
            n247 = Close File(refnum=w374, error in=w373) -> ()  [unwired: 2 out]
          }
        }
      }
      event "运行间隔", "多参数运行间隔": Mouse Down {
        n248 = event-data() -> ("CtlRef"=w385:refnum<vi>)  [unwired: 1 in, 7 out]
        n249 = property class="DigNum (严格)"(reference=w385) -> (reference out=w384:refnum<vi>, "Value"=w383:i16)  [unwired: 1 in, 1 out]
        n250 = call "数字键盘.vi"("OldNumber"=w383) -> ("NewNumber"=w382:sgl)
        n251 = property class="DigNum (严格)"(reference=w384, "Val(Sgnl)"=w382) -> ()  [unwired: 1 in, 2 out]
      }
      event "添加防火墙": Value Change {
        n252 = event-data() -> ()  [unwired: 1 in, 6 out]
        n253 = flat-sequence {
          frame #0 {
            # "添加防火墙规则"
            n254 = call "add application firewall rule.vi"() -> ()  [unwired: 12 in]
            n255 = call "add NI PSP Service Locator firewall.vi"() -> ()  [unwired: 12 in]
          }
        }
      }
      event "流量阈值": Mouse Down {
        n256 = event-data() -> ("CtlRef"=w389:refnum<vi>)  [unwired: 1 in, 7 out]
        n257 = property class="DigNum (严格)"(reference=w389) -> (reference out=w388:refnum<vi>, "Value"=w387:dbl)  [unwired: 1 in, 1 out]
        n258 = call "数字键盘.vi"("OldNumber"=w387) -> ("NewNumber"=w386:sgl)
        n259 = property class="DigNum (严格)"(reference=w388, "Val(Sgnl)"=w386) -> ()  [unwired: 1 in, 2 out]
      }
      event "时间阈值": Mouse Down {
        n260 = event-data() -> ("CtlRef"=w393:refnum<vi>)  [unwired: 1 in, 7 out]
        n261 = property class="DigNum (严格)"(reference=w393) -> (reference out=w392:refnum<vi>, "Value"=w391:u16)  [unwired: 1 in, 1 out]
        n262 = call "数字键盘.vi"("OldNumber"=w391) -> ("NewNumber"=w390:sgl)
        n263 = property class="DigNum (严格)"(reference=w392, "Val(Sgnl)"=w390) -> ()  [unwired: 1 in, 2 out]
      }
      event "开机启动": Value Change {
        n264 = event-data() -> ("NewVal"=w395:bool)  [unwired: 1 in, 5 out]
        n265 = call <vilib>:"Application Directory.vi"() -> ("Application Directory"=w394:path)
        n266 = case shown="假" w395 {
          tunnel: w394 -> [_ w400]
          frame False {
            n267 = call "删除启动项.vi"() -> ("删除标记"=w396:bool)  [unwired: 10 in, 1 out]
            n268 = case shown="假" w396 {
              frame False {
                n269 = local write "开机启动"(TRUE ("开机启动")) -> ()
                n270 = One Button Dialog(message="启动项删除失败" ("消息")) -> ()  [unwired: 1 in, 1 out]
              }
              frame True {
              }
            }
          }
          frame True {
            n271 = call "添加启动项.vi"("启动文件路径"=w400) -> ("添加成功标记"=w399:bool)  [unwired: 9 in, 1 out]
            n272 = case shown="假" w399 {
              frame False {
                n273 = local write "开机启动"(FALSE ("开机启动")) -> ()
                n274 = One Button Dialog(message="启动项添加失败" ("消息")) -> ()  [unwired: 1 in, 1 out]
              }
              frame True {
              }
            }
          }
        }
      }
      event "首页显示设置": Value Change {
        n275 = event-data() -> ()  [unwired: 1 in, 6 out]
        n276 = call "首页显示设置.vi"() -> ()  [unwired: 12 in]
      }
      event "短信报警设置": Value Change {
        n277 = event-data() -> ()  [unwired: 1 in, 6 out]
        n278 = invoke class="VI" method="FP.Open"(reference=w405, "Activate"=TRUE ("激活？"), "State"=T11."Standard" ("状态")) -> ()  [unwired: 2 in, 5 out]
      }
      event "微信关注扫码": Value Change {
        n279 = event-data() -> ()  [unwired: 1 in, 6 out]
        n280 = call "创建参数二维码.vi"() -> ()  [unwired: 12 in]
      }
      event "站点配置": Value Change {
        n281 = event-data() -> ()  [unwired: 1 in, 6 out]
        n282 = call "站点信息配置.vi"() -> ()  [unwired: 12 in]
      }
      event "布尔": Mouse Down {
        n283 = event-data() -> ("CtlRef"=w407:refnum<vi>)  [unwired: 1 in, 7 out]
        n284 = property class="Bool (严格)"(reference=w407) -> ("Value"=w406:bool)  [unwired: 1 in, 2 out]
        n285 = case shown="假" w406 {
          tunnel: [w409 _] -> w408
          frame False {
            n286 = call "数字密码键盘.vi"() -> ("NewNumber"=w409:sgl)  [unwired: 1 in]
          }
          frame True {
          }
        }
        n287 = local write "输入密码"(w408) -> ()
      }
    }
  }
  n288 = Index Array(array=w47) -> (element=w49:path)  [unwired: 1 in]
  n289 = Build Array("主机" ("section"), "用户" ("section"), "密码" ("key"), "远程路径" ("key"), "下载文件名" ("key"), "软件版本" ("key")) -> (w27:string[])
  n290 = Build Path(base path=w28, name or relative path="set.ini" ("名称或相对路径")) -> (appended path=w52:path)
  n291 = call <vilib>:"FileVersionInfo.vi"("error in (no error)"=w45, "Application Path in"=w49) -> ("error out"=w42:errorcluster, "File Version Info"=w43:string)  [unwired: 6 in, 2 out]
  n292 = call <userlib>:"Abort Balloon Engine.vi"("error in (no error)"=w22, "SmartBalloon Engine Reference"=w23) -> ("error out"=w20:errorcluster)  [unwired: 9 in]
  n293 = call <vilib>:"Simple Error Handler.vi"("error in (no error)"=w20) -> ()  [unwired: 4 in, 5 out]
  n294 = call "配置文件read.vi"("error in (no error)"=w42, "configuration file path"=w52, "键数组"=w27, "段"=w53) -> ("error out"=w51:errorcluster, "section exists?"=w54:bool, "updateconfiguration"=w50:T1)  [unwired: 5 in]
  n295 = Concatenate Strings("V" ("字符串"), w43) -> (w41:string)
  n296 = case shown="假" w54 {
    tunnel: w27 -> [w421 w425]
    tunnel: w53 -> [w420 w429]
    tunnel: w52 -> [w419 w423]
    tunnel: w51 -> [_ w424]
    tunnel: [w418 w422] -> w40
    tunnel: w50 -> [w412 w428]
    tunnel: [w410 w426] -> w26
    tunnel: w41 -> [w411 w427]
    frame False {
      # "赋初值"
      n297 = Bundle By Name(cluster=w412, "主机"="27.154.58.30" ("key"), "用户"="update", "密码"="std23506", "远程路径"="固定站系统_固定站_V4\\一体化水质自动监测系统.exe", "下载文件名"="一体化水质自动监测系统.exe", "软件版本"=w411) -> (w410:T1)
      n298 = call "配置文件write.vi"("updateconfiguration"=w410, "configuration file path"=w419, "键数组"=w421, "段"=w420) -> ("error out"=w418:errorcluster)  [unwired: 7 in]
    }
    frame True {
      # "读取本地保存"
      n299 = Bundle By Name(cluster=w428, "软件版本"=w427) -> (w426:T1)
      n300 = call "配置文件write.vi"("updateconfiguration"=w426, "error in (no error)"=w424, "configuration file path"=w423, "键数组"=w425, "段"=w429) -> ("error out"=w422:errorcluster)  [unwired: 6 in]
    }
  }
  n301 = global write "update全局.vi" "updateconfiguration"(w26) -> ()
  n302 = while {
    tunnel: [w430] -> _
    tunnel: w40 -> [_]
    stop <- FALSE stop-if-true
    n303 = event shown="[2] \"更新\": 值改变" {
      selector: _ -> [_ _ _]
      dyn-events: _ -> [_ _ _]
      timeout: 1000 -> [_ _ _]
      tunnel: [_ w441 _] -> w430
      event Timeout {
        n304 = event-data() -> ()  [unwired: 1 in, 3 out]
        n305 = local read "updateconfiguration"() -> (w433:T1)
        n306 = global write "update全局.vi" "updateconfiguration"(w433) -> ()
      }
      event "updateconfiguration": Value Change {
        n307 = event-data() -> ()  [unwired: 1 in, 6 out]
        n308 = call <vilib>:"Application Directory.vi"() -> ("Application Directory"=w444:path)
        n309 = Build Path(base path=w444, name or relative path="update\\data\\set.ini" ("名称或相对路径")) -> (appended path=w442:path)
        n310 = Build Array("主机" ("section"), "用户" ("section"), "密码" ("key"), "远程路径" ("key"), "下载文件名" ("key"), "软件版本" ("key")) -> (w434:string[])
        n311 = call "配置文件write.vi"("configuration file path"=w442, "键数组"=w434, "段"="应用程序交互" ("section")) -> ("error out"=w441:errorcluster)  [unwired: 8 in]
      }
      event "更新": Value Change {
        n312 = event-data() -> ()  [unwired: 1 in, 6 out]
        n313 = call "FTP自动升级更新main.vi"() -> ()  [unwired: 12 in]
      }
    }
  }
  n314 = local write "updateconfiguration"(w26) -> ()
